vi "Part 1.vi"(11 "Input":string) -> (3 "Output":i64)   [LabVIEW 2021]
uses:
  <userlib>/_OpenG.lib/string/string.llb/Convert EOLs (String)__ogtk.vi
panel:
  out "Output String":string
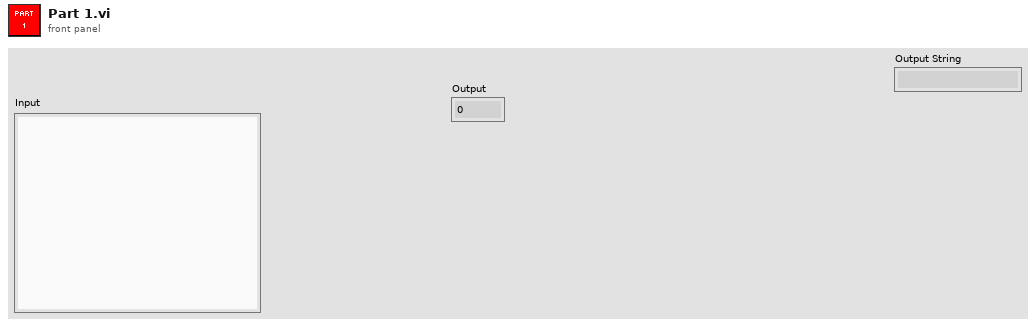
[diagram p1: front panel]
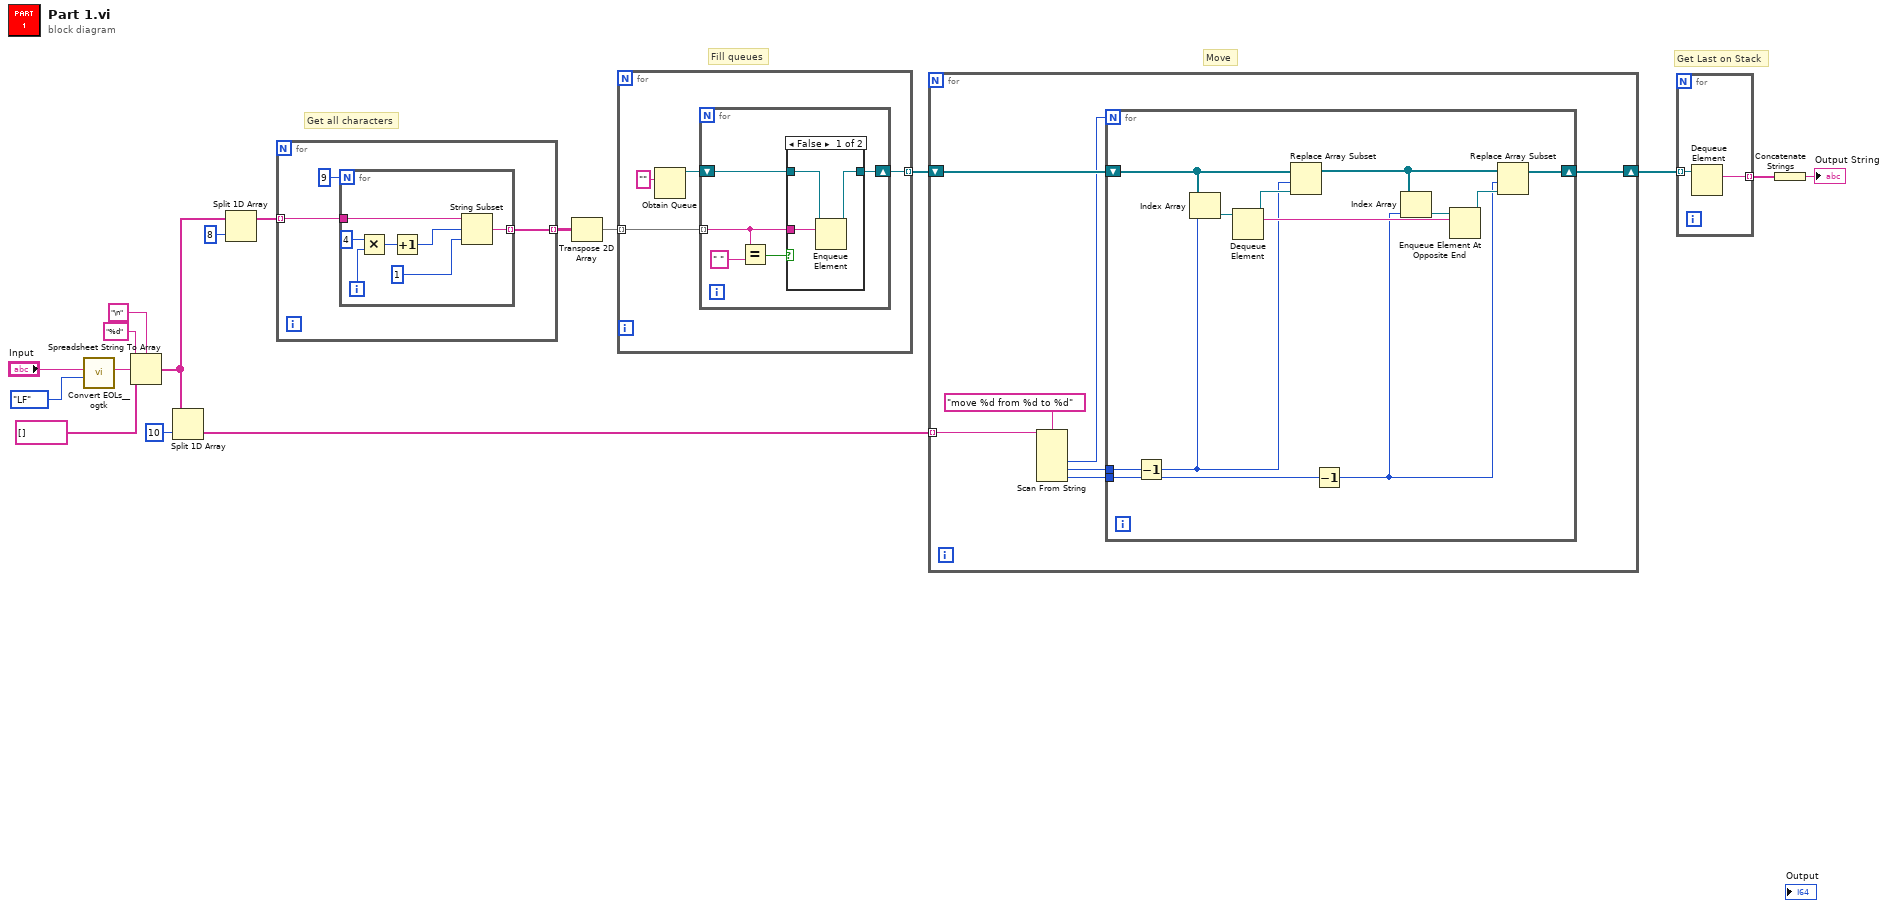
[diagram p0: block diagram]
diagram:
  # "Get Last on Stack"
  # "Move"
  # "Fill queues"
  # "Get all characters"
  n1 = call-poly <userlib>:"Convert EOLs__ogtk.vi"("Convert to:"=enum16{"CR", "LF", "CRLF"}."LF", "String in"="Input") -> ("String out"=w14:string)  [unwired: 9 in]
  n2 = Spreadsheet String To Array(delimiter (Tab)="\n", format string="%d", spreadsheet string=w14, array type (2D Dbl)=string[] []) -> (array=w10:string[])
  n3 = Split 1D Array(array=w10, index=10) -> (second subarray=w6:string[])  [unwired: 1 out]
  n4 = Split 1D Array(array=w10, index=8) -> (first subarray=w9:string[])  [unwired: 1 out]
  n5 = for {
    tunnel: w9 -> [w20] mode=indexing
    tunnel: [w18] -> w8 mode=indexing
    n6 = for {
      N: 9 -> [_]
      tunnel: w20 -> [w27]
      tunnel: [w24] -> w18 mode=indexing
      i -> [w26]
      n7 = Multiply(x=4, y=w26) -> (x*y=w23:i32)
      n8 = Increment(x=w23) -> (x+1=w22:i32)
      n9 = String Subset(string=w27, offset (0)=w22, length (rest)=1 ("length (rest)")) -> (substring=w24:string)
    }
  }
  n10 = Transpose 2D Array(2D array=w8) -> (transposed array=w7:string[][])
  n11 = for {
    tunnel: w7 -> [w30] mode=indexing
    tunnel: [w28] -> w5 mode=indexing
    n12 = Obtain Queue(element data type="") -> (queue out=w29:refnum<queue>)  [unwired: 4 in, 2 out]
    n13 = for {
      tunnel: w30 -> [w33] mode=indexing
      shift-right: [w35] -> w28
      shift-left: w29 -> [w36]
      n14 = Equal?(x=w33, y=" ") -> (x = y?=w34:bool)
      n15 = case shown="False" w34 {
        tunnel: w36 -> [w39 w40]
        tunnel: [w38 w40] -> w35
        tunnel: w33 -> [w37 _]
        frame False {
          n16 = Enqueue Element(queue=w39, element=w37) -> (queue out=w38:refnum<queue>)  [unwired: 2 in, 2 out]
        }
        frame True {
        }
      }
    }
  }
  n17 = for {
    tunnel: w6 -> [w47] mode=indexing
    shift-right: [w43] -> w4
    shift-left: w5 -> [w46]
    n18 = Scan From String(format string="move %d from %d to %d", input string=w47) -> (output 1=w42:i32, output 2=w45:i32, output 3=w44:i32)  [unwired: 5 in, 3 out]
    n19 = for {
      N: w42 -> [_]
      tunnel: w45 -> [w57]
      tunnel: w44 -> [w53]
      shift-right: [w52] -> w43
      shift-left: w46 -> [w58]
      n20 = Decrement(x=w57) -> (x-1=w48:i32)
      n21 = Index Array(array=w58, index=w48) -> (element=w59:refnum<queue>)
      n22 = Dequeue Element(queue=w59) -> (queue out=w51:refnum<queue>, element=w50:string)  [unwired: 2 in, 2 out]
      n23 = Replace Array Subset(array=w58, new element=w51, index=w48) -> (w55:refnum<queue>[])
      n24 = Decrement(x=w53) -> (x-1=w49:i32)
      n25 = Index Array(array=w55, index=w49) -> (element=w56:refnum<queue>)
      n26 = Enqueue Element At Opposite End(queue=w56, element=w50) -> (queue out=w54:refnum<queue>)  [unwired: 2 in, 2 out]
      n27 = Replace Array Subset(array=w55, new element=w54, index=w49) -> (w52:refnum<queue>[])
    }
  }
  n28 = for {
    tunnel: w4 -> [w61] mode=indexing
    tunnel: [w60] -> w3 mode=indexing
    n29 = Dequeue Element(queue=w61) -> (element=w60:string)  [unwired: 2 in, 3 out]
  }
  n30 = Concatenate Strings(w3) -> (→"Output String":string)
